vi "Write Averager.vi"(8 "error in (no error)":errorcluster, 10 "Averager":refnum<class "Roughness Averager.lvclass">, 11 "Video Processor in":refnum<class "Video Cam Processor.lvclass">) -> (0 "error out":errorcluster, 3 "Video Processor out":refnum<class "Video Cam Processor.lvclass">)   [LabVIEW 2018, in "Video Cam Processor.lvclass"]
uses:
  Video Cam Processor.lvclass
  Roughness Averager/Roughness Averager.lvclass
  Video Cam Processor.lvclass/Video Cam Processor.ctl
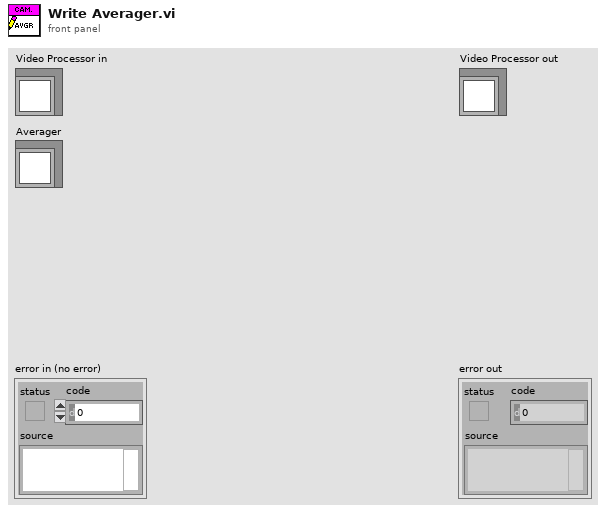
[diagram p1: front panel]
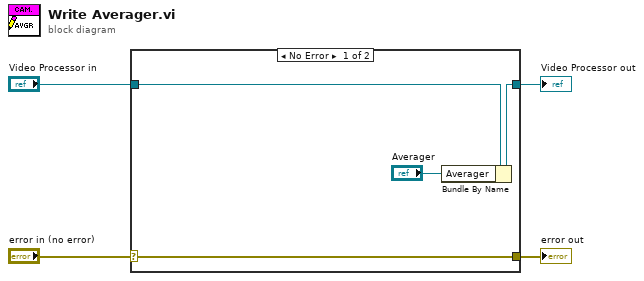
[diagram p0: block diagram]
diagram:
  n1 = case shown="No Error" "error in (no error)" {
    selector: "error in (no error)" -> [w8 w9]
    tunnel: [w8 w9] -> w3
    tunnel: [w6 w10] -> w1
    tunnel: "Video Processor in" -> [w7 w10]
    frame No Error {
      n2 = Bundle By Name(cluster=w7, "Averager"="Averager") -> (w6:refnum<class "Video Cam Processor.lvclass">)
    }
    frame Error {
    }
  }
  "error out" <- w3
  "Video Processor out" <- w1
